vi "OUINON.vi"(8 "errin":errorcluster, 11 "image":string) -> (0 "error out":errorcluster caption="errout", 3 "OUI/NON":bool)   [LabVIEW 2020]
uses:
  <userlib>/FGV/FGV.ctl
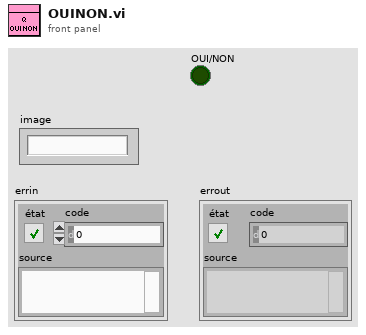
[diagram p1: front panel]
types:
  T1 = typedef "FGV.ctl" = enum16{"GET", "SET", "RAZ"}
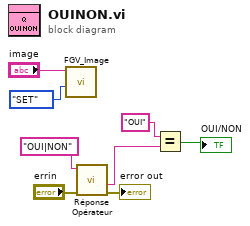
[diagram p0: block diagram]
diagram:
  n1 = call <userlib>:"FGV_Image.vi"("Énum"=FGV."SET", "IN"="image") -> ()  [unwired: 9 in, 1 out]
  n2 = call "Réponse Opérateur.vi"("errin"="errin", "expression régulière"="OUI|NON") -> ("errout"=→"error out":errorcluster, "toute l'expression"=w2:string)  [unwired: 7 in, 1 out]
  n3 = Equal?(x="OUI" ("y"), y=w2) -> (x = y?=→"OUI/NON":bool)
